vi "Q8381 QRY SPAN_SPAN.vi"(0 "VISA resource name":refnum<visa-resource-name>, 1 "GPIB Address":u16=8 max=31 step=1) -> (2 "GPIB Status":bool, 3 "Span data":string, 4 "Span value":dbl format="%.5e")   [LabVIEW 2017]
panel:
  # "Query  SPAN"
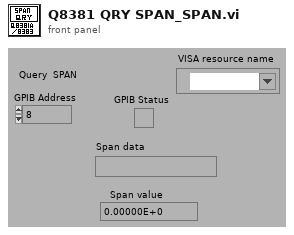
[diagram p1: front panel]
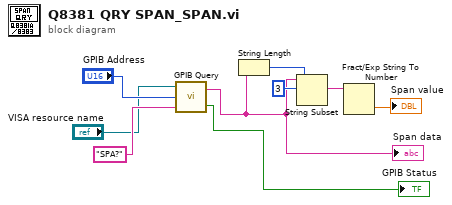
[diagram p0: block diagram]
diagram:
  n1 = call "GPIB Query.vi"("Command String"="SPA?", "Address"="GPIB Address", "VISA resource name"="VISA resource name") -> ("Error"=→"GPIB Status":bool, "Query Data"=w3:string)
  "Span data" <- w3
  n2 = String Length(string=w3) -> (length=w8:i32)
  n3 = String Subset(string=w3, offset (0)=3, length (rest)=w8) -> (substring=w7:string)
  n4 = Fract/Exp String To Number(string=w7) -> (number=→"Span value":dbl)  [unwired: 3 in, 1 out]
